vi "DIO64 Out Start.vi"(0 "board in":u16 format="%.0x", 11 "error in (no error)":errorcluster) -> (4 "board out":u16 format="%.0x", 15 "error out":errorcluster)   [LabVIEW 2012]
doc: "DIO64 Out Start writes the data in the output buffer to the DIO-64 ports. This VI should only be used for output-only operation. For combined input and output operation, DIO64 In Start.vi will start both input and output.\n\nCopyright (c) 2002 Viewpoint Systems Inc. All Rights Reserved"
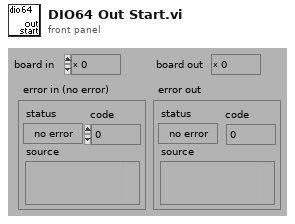
[diagram p1: front panel]
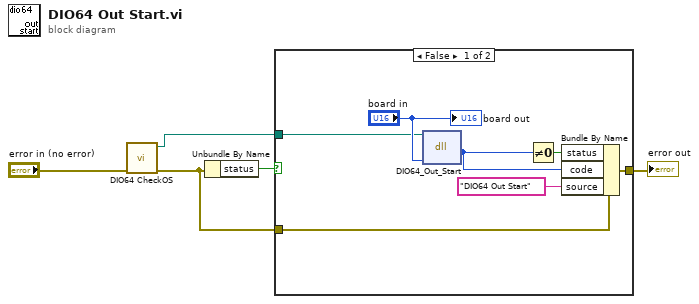
[diagram p0: block diagram]
diagram:
  n1 = call "DIO64 CheckOS.vi"("error in"="error in (no error)") -> ("error out"=w2:errorcluster, "path in"=w1:path)  [unwired: 9 in]
  n2 = Unbundle By Name(w2) -> ("status"=w5:bool)
  n3 = case shown="False" w5 {
    tunnel: w2 -> [w10 w13]
    tunnel: [w9 w13] -> w4
    tunnel: w1 -> [w6 _]
    frame False {
      n4 = dll-call lib="C:/DIO64Visa/DLL/DIO64_Visa32/Debug/DIO64_Visa32.dll" fn="DIO64_Out_Start"(path in=w6, "board"="board in") -> ("return type"=w12:i32)  [unwired: 3 in, 2 out]
      n5 = Not Equal To 0?(x=w12) -> (x != 0?=w11:bool)
      n6 = Bundle By Name(cluster=w10, "status"=w11, "code"=w12, "source"="DIO64 Out Start") -> (w9:errorcluster)
      "board out" <- "board in"
    }
    frame True {
    }
  }
  "error out" <- w4
